vi "RT Driver VI.vi"(7 "Operation":T1, 11 "Device Reference in":T2 format="%.0x") -> (0 "Error Code":i32)   [LabVIEW 2015, in "OPC UA Client Engine.lvlib"]
uses:
  OPC UA Client Engine.lvlib
  <vilib>/NI Veristand/Custom Device API/Custom Device Item Ref.ctl
  <vilib>/NI Veristand/Custom Device API/Hardware Interface Driver VI Operation.ctl
  Types/Main.StateVariables.ctl
  Types/Poll.Parameters.ctl
  Shared/Compiled.Settings.ctl
  Shared/OPCConnection.Properties.ctl
  Shared/Poll.ListProperties.ctl
  <vilib>/NI Veristand/Custom Device API/Data Reference.ctl
  Shared/Tag.WriteProperties.Info.ctl
  Shared/Tags.ReadWriteRefs.ctl
  <vilib>/NI Veristand/Custom Device API/Custom Device Target Type.ctl
  SubVIs/Error Handling API/Controls/Error Handling Cluster.ctl
  <vilib>/NI Veristand/Custom Device API/NI VeriStand - Set Channel Value by Data Reference.vi
  <vilib>/NI Veristand/Custom Device API/NI VeriStand - Get Channel Value by Data Reference.vi
  SubVIs/Error Handling API/Display and Log Process.vi
  Shared/Constants.vi
  <vilib>/NI Veristand/Custom Device Tools/Custom Device Utility Library/NI VeriStand - Print Debug String.vi
  <vilib>/NI Veristand/Custom Device API/NI VeriStand - Get Item Data.vi
  <vilib>/NI Veristand/Custom Device API/NI VeriStand - Get Target Type.vi
  <vilib>/NI Veristand/Custom Device API/NI VeriStand - Get Item Property.vi
  <vilib>/NI Veristand/Custom Device API/Get Item Property (Variant).vi
  <vilib>/NI Veristand/Custom Device API/Global Data Refs.vi
  SubVIs/Inline Async API/Close Async VIs.vi
  <vilib>/NI Veristand/Custom Device API/Custom Device API.lvlib
  Shared/OPC UA Client Shared.lvlib
  SubVIs/Inline Async API/Inline Async API.lvlib
  SubVIs/Error Handling API/Error Handling API.lvlib
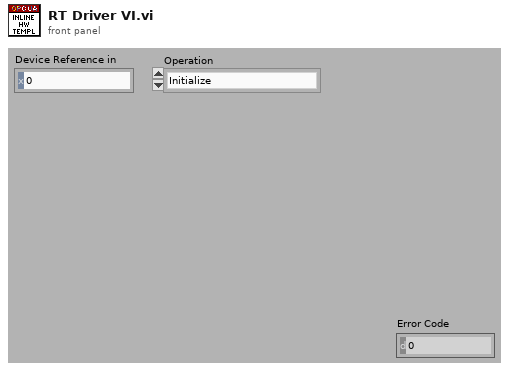
[diagram p1: front panel]
types:
  T1 = typedef "Custom Device API.lvlib/Hardware Interface Driver VI Operation.ctl" = enum16{"Initialize", "Start", "Read Data from HW", "Write Data to HW", "Close"}
  T2 = typedef "Custom Device API.lvlib/Custom Device Item Ref.ctl" = u64
  T3 = typedef "OPC UA Client Engine.lvlib/Main.StateVariables.ctl" = cluster{"Parameters":T4, "VI Refs":refnum<vi>[], "Error Refs":T12}
  T4 = typedef "OPC UA Client Engine.lvlib/Poll.Parameters.ctl" = cluster{"Settings":T5, "WriteData":refnum<k33>, "ReadData":refnum<k33>, "StatusData":refnum<k33>, "WriteUpdate":refnum<k33>, "ReadUpdate":refnum<k33>, "Target Type":T11}
  T5 = typedef "OPC UA Client Shared.lvlib/Compiled.Settings.ctl" = cluster{"Connection.Properties":T6, "PollEngine.Settings":T7[], "StatusRefs":cluster{"Chan Refs":T8[], "Values Array":dbl[]}, "LUT":variant, "Write Locations":T9[], "TotalTags":u32, "Data Refs":T10}
  T6 = typedef "OPC UA Client Shared.lvlib/OPCConnection.Properties.ctl" = cluster{"Server IP Address":string, "Server Port":u16, "Message Mode":enum16{"None", "Sign", "Sign and Encrypt"}, "Security":enum16{"Basic256", "Basic128Rsa15"}, "User Name":string, "Password":string, "Client Certificate":path, "Server Certificate":path, "Server Certificate (RT)":path, "Client Certificate (RT)":path}
  T7 = typedef "OPC UA Client Shared.lvlib/Poll.ListProperties.ctl" = cluster{"Poll Rate":dbl, "Tags":string[]}
  T8 = typedef "Custom Device API.lvlib/Data Reference.ctl" = i32
  T9 = typedef "OPC UA Client Shared.lvlib/Tag.WriteProperties.Info.ctl" = cluster{"Path":string, "Offset":i32, "Length":i32, "DataType":u32}
  T10 = typedef "OPC UA Client Shared.lvlib/Tags.ReadWriteRefs.ctl" = cluster{"Read Refs":T8[], "Read Values":dbl[], "Read?":bool[], "Access":enum8{"Null", "Read", "Write", "Read&Write"}[], "Write Refs":T8[], "Write Values":dbl[], "Write?":bool[], "Write Only Location":u32, "Write? Reset":bool[]}
  T11 = typedef "Custom Device API.lvlib/Custom Device Target Type.ctl" = enum16{"PharLap", "VxWorks", "Windows"}
  T12 = typedef "OPC UA Client Engine.lvlib/Error Handling API.lvlib/Error Handling Cluster.ctl" = cluster{"Error Process Q":refnum<queue>, "Process Qs":refnum<queue>[]}
  T13 = cluster{"Chan Refs":T8[], "Previous Chan Values":dbl[]}
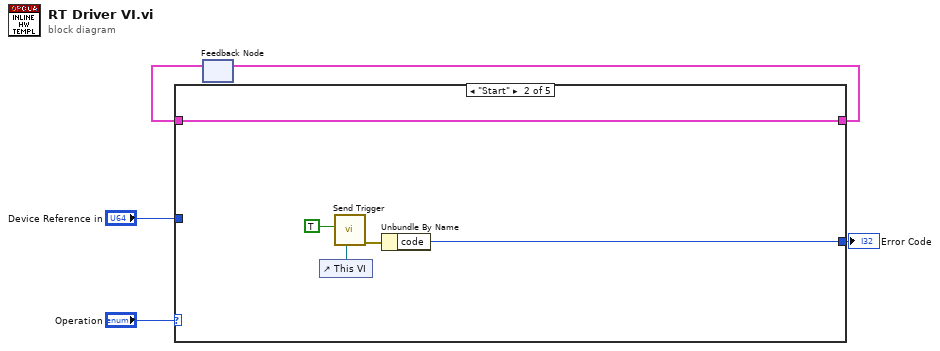
[diagram p0: block diagram]
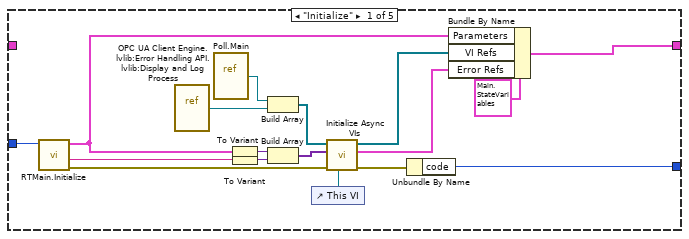
[diagram p2: hidden frame]
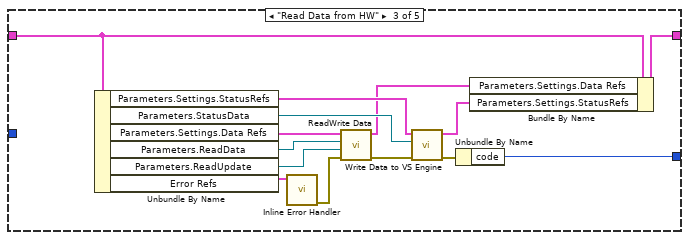
[diagram p3: hidden frame]
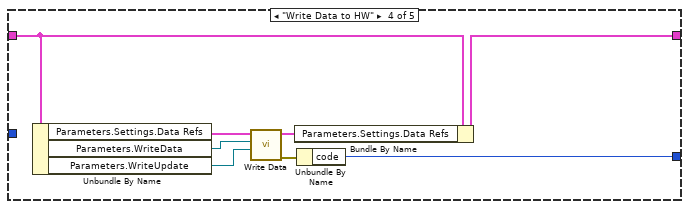
[diagram p4: hidden frame]
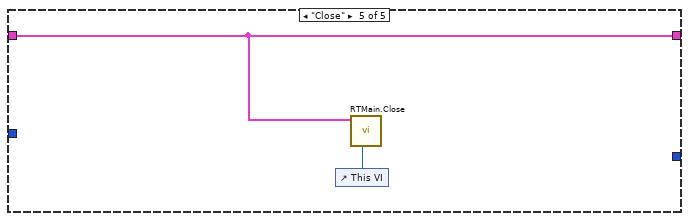
[diagram p5: hidden frame]
diagram:
  n1 = feedback #1() -> (w3:T3)  [unwired: 1 out]
  n2 = case shown="\"Start\"" "Operation" {
    tunnel: [w20 w26 w39 w48 w51] -> w4
    tunnel: w3 -> [_ w26 w40 w49 w51]
    tunnel: "Device Reference in" -> [w21 _ _ _ _]
    tunnel: [w22 w27 w41 w47 _] -> w1
    frame "Initialize" {
      n3 = call "RTMain.Initialize.vi"("Device Reference in"=w21) -> ("error out"=w19:errorcluster, "Name"=w14:string, "Parameters"=w15:T4)  [unwired: 8 in]
      n4 = vi-ref "OPC UA Client Engine.lvlib:Error Handling API.lvlib:Display and Log Process.vi"() -> (w7:refnum<vi>)
      n5 = vi-ref "Poll.Main.vi"() -> (w8:refnum<vi>)
      n6 = To Variant(anything=w15) -> (Variant=w12:variant)
      n7 = To Variant(anything=w14) -> (Variant=w6:variant)
      n8 = Build Array(w8, w7) -> (w9:refnum<vi>[])
      n9 = Build Array(w12, w6) -> (w10:variant[])
      n10 = control-ref of="This VI"() -> (w11:refnum<vi>)
      n11 = call "Initialize Async VIs.vi"("VI in"=w11, "error in (no error)"=w19, "Async VI Parameters"=w10, "Async VI Refs"=w9) -> ("error out"=w18:errorcluster, "Error Handling Refs"=w13:T12, "Async VI Refs out"=w17:refnum<vi>[])  [unwired: 5 in]
      n12 = Unbundle By Name(w18) -> ("code"=w22:i32)
      n13 = Bundle By Name(cluster=T3 {"Parameters"={"Settings"={"Connection.Properties"={"Server IP Address"="", "Server Port"=0, "Message Mode"=enum."None", "Security"=enum."Basic256", "User Name"="", "Password"="", "Client Certificate"=path "", "Server Certificate"=path "", "Server Certificate (RT)"=path "", "Client Certificate (RT)"=path ""}, "PollEngine.Settings"=[], "StatusRefs"={"Chan Refs"=[], "Values Array"=[]}, "LUT"=variant, "Write Locations"=[], "TotalTags"=0, "Data Refs"={"Read Refs"=[], "Read Values"=[], "Read?"=[], "Access"=[], "Write Refs"=[], "Write Values"=[], "Write?"=[], "Write Only Location"=0, "Write? Reset"=[]}}, "WriteData"=refnum, "ReadData"=refnum, "StatusData"=refnum, "WriteUpdate"=refnum, "ReadUpdate"=refnum, "Target Type"=enum."PharLap"}, "VI Refs"=[], "Error Refs"={"Error Process Q"=refnum, "Process Qs"=[]}}, "Parameters"=w15, "VI Refs"=w17, "Error Refs"=w13) -> (w20:T3)
    }
    frame "Start" {
      n14 = control-ref of="This VI"() -> (w24:refnum<vi>)
      n15 = call "Send Trigger.vi"("Parent VI"=w24, "notification"=TRUE) -> ("error out"=w23:errorcluster)  [unwired: 9 in]
      n16 = Unbundle By Name(w23) -> ("code"=w27:i32)
    }
    frame "Read Data from HW" {
      n17 = Unbundle By Name(w40) -> ("Parameters.Settings.StatusRefs"=w33:cluster{"Chan Refs":T8[], "Values Array":dbl[]}, "Parameters.StatusData"=w34:refnum<k33>, "Parameters.Settings.Data Refs"=w31:T10, "Parameters.ReadData"=w35:refnum<k33>, "Parameters.ReadUpdate"=w28:refnum<k33>, "Error Refs"=w36:T12)
      n18 = call "Inline Error Handler.vi"("Error Handling Cluster"=w36) -> ("error out"=w29:errorcluster)  [unwired: 10 in]
      n19 = call "ReadWrite Data.vi"("error in"=w29, "ReadUpdate"=w28, "Write to VS Engine FIFO"=w35, "Data Refs"=w31) -> ("error out"=w32:errorcluster, "Data Refs"=w30:T10)  [unwired: 5 in, 1 out]
      n20 = call "Write Data to VS Engine.vi"("error in"=w32, "Write to VS Engine FIFO"=w34, "Channel Pairs"=w33) -> ("error out"=w38:errorcluster, "Channel Pairs Out"=w37:T13)  [unwired: 6 in, 1 out]
      n21 = Unbundle By Name(w38) -> ("code"=w41:i32)
      n22 = Bundle By Name(cluster=w40, "Parameters.Settings.Data Refs"=w30, "Parameters.Settings.StatusRefs"=w37) -> (w39:T3)
    }
    frame "Write Data to HW" {
      n23 = Unbundle By Name(w49) -> ("Parameters.Settings.Data Refs"=w46:T10, "Parameters.WriteData"=w44:refnum<k33>, "Parameters.WriteUpdate"=w43:refnum<k33>)
      n24 = call "Write Data.vi"("WriteUpdate"=w43, "Read from VS Engine FIFO"=w44, "Data Refs"=w46) -> ("error out"=w42:errorcluster, "Data Refs"=w45:T10)  [unwired: 7 in]
      n25 = Bundle By Name(cluster=w49, "Parameters.Settings.Data Refs"=w45) -> (w48:T3)
      n26 = Unbundle By Name(w42) -> ("code"=w47:i32)
    }
    frame "Close" {
      n27 = control-ref of="This VI"() -> (w50:refnum<vi>)
      n28 = call "RTMain.Close.vi"("VI in"=w50, "cluster"=w51) -> ()  [unwired: 10 in]
    }
  }
  "Error Code" <- w1
  n29 = feedback-in #1(w4) -> ()
